vi "hacercirculo.vi"() -> ()   [LabVIEW 2016]
panel:
  out "Waveform Graph 2":dbl[](graph)
  out "Waveform Graph":dbl[](graph)
  out "XY Graph":cluster{dbl[], dbl[]}(graph)
  in  "n":dbl
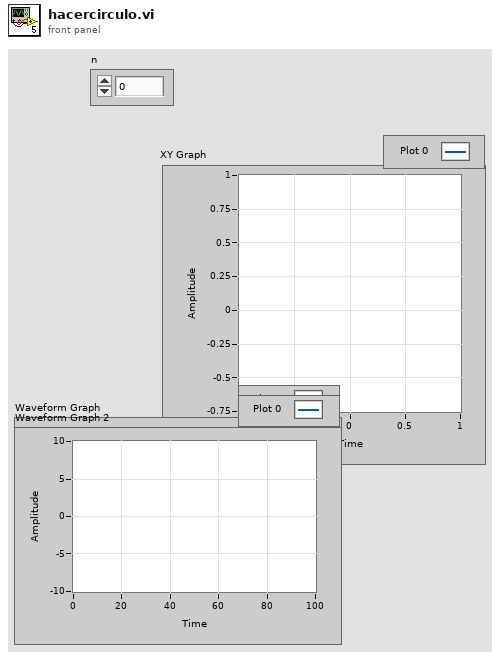
[diagram p1: front panel]
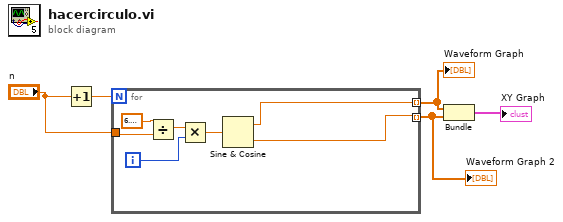
[diagram p0: block diagram]
diagram:
  n1 = Increment(x="n") -> (x+1=w3:dbl)
  n2 = for {
    N: w3 -> [_]
    tunnel: "n" -> [w11]
    tunnel: [w7] -> w2 mode=indexing
    tunnel: [w6] -> w1 mode=indexing
    i -> [w9]
    n3 = Divide(x=6.283185307179586, y=w11) -> (x/y=w10:dbl)
    n4 = Multiply(x=w10, y=w9) -> (x*y=w8:dbl)
    n5 = Sine & Cosine(0:w8) -> (1:w7:dbl, 2:w6:dbl)
  }
  "Waveform Graph" <- w2
  "Waveform Graph 2" <- w1
  n6 = Bundle(w2, w1) -> (→"XY Graph":cluster{dbl[], dbl[]})  [unwired: 1 in]
